vi "PH_Stepmotor_BaseClass.ProcCases.vi"(0 "i ref in":refnum<vi>, 1 "selector":string, 2 "Data":T1, 3 "call cluster":T2={"Object"="", "Selector"="", "CallType"=enum."synchronous", "Async Object"="", "Async Selector"="", "Data Descriptor"="", "Data"=[], "Error #"=0, "Expire"=0}, 5 "error in":errorcluster) -> (14 "i ref out":refnum<vi>, 17 "answer cluster":T2={"Object"="", "Selector"="", "CallType"=enum."synchronous", "Async Object"="", "Async Selector"="", "Data Descriptor"="", "Data"=[], "Error #"=0, "Expire"=0}, 19 "error out":errorcluster)   [LabVIEW 2014, in "PH_Stepmotor_BaseClass.lvlib"]
doc: "This method is called by a process from within the default case in the event loop. The methods of a class that are linked to events will be called from THIS method. Add your code here."
uses:
  PH_Stepmotor_BaseClass.lvlib
  CSCore/CSSystem/CoreDefs/CoreDefs.call_type.ctl
  CSCore/BaseProcess/BaseProcess.descriptor string definition.ctl
  CSCore/CSSystem/CoreDefs/CoreDefs.rawDataType.ctl
  PH_PSDBWriter/PH_PSDBWriter.Thread Commands.ctl
  PH_Stepmotor_BaseClass.Axis Settings.ctl
  PH_Stepmotor_BaseClass.Motor Type.ctl
  PH_Stepmotor_BaseClass.Axis Direction.ctl
  CSCore/CSSystem/CoreLib/CoreLib.string 2 byte array.vi
  CSCore/CSSystem/CoreLib/CoreLib.byte array 2 short.vi
  CSCore/CSSystem/CoreLib/CoreLib.byte array 2 int.vi
  CSCore/CSSystem/CoreLib/CoreLib.byte array 2 double.vi
  CSCore/CSSystem/CoreLib/CoreLib.byte array 2 string.vi
  CSCore/CSSystem/CoreLib/CoreLib.lvlib
  CSCore/BaseProcess/BaseProcess.lvlib
  PH_PSDBWriter/PH_PSDBWriter.lvlib
  CSCore/CAEObj/CAEObj.lvlib
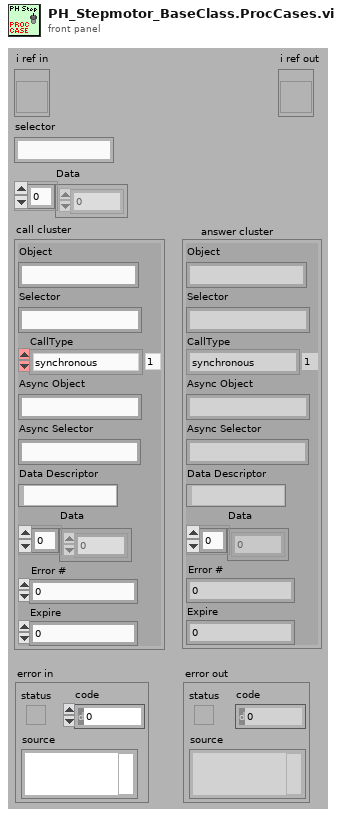
[diagram p1: front panel]
types:
  T1 = typedef "CoreDefs.rawDataType.ctl" = i8[]
  T2 = typedef "CoreDefs.call_type.ctl" = cluster{"Object":string, "Selector":string, "CallType":enum16{"simple", "synchronous", "asynchronous"}, "Async Object":string, "Async Selector":string, "Data Descriptor":T3, "Data":T1, "Error #":i32, "Expire":u32}
  T3 = typedef "BaseProcess.lvlib/BaseProcess.descriptor string definition.ctl" = string
  T4 = typedef "PH_Stepmotor_BaseClass.lvlib/PH_Stepmotor_BaseClass.Axis Settings.ctl" = cluster{"Sign change":bool, "Width":dbl, "Calibration":dbl, "Unit":string, "Motor Type":T5, "Unit Width":string, "Unit CF":string}
  T5 = typedef "PH_Stepmotor_BaseClass.lvlib/PH_Stepmotor_BaseClass.Motor Type.ctl" = enum16{"Unspecific", "OWIS 49.120.2633", "OWIS 49.060.1033", "OWIS 43.040.2558", "Diamond Motion 2200 series", "OWIS 49.120.266B.MV6", "Calorimeter", "Linear Stage 1", "MICOS VT-80", "MICOS VT-80 S", "Standa Rotstage nt0.95A", "PUF RA 320.200", "PUF RA 800.200", "PUF RA 800.400", "PUF RA 400.50", "1324.nn.800.50", "1324.n9c.800.50", "1324.nn.320.200", "1324.nn.400.200", "1324.nn.800.200", "1324.nn.400.50", "1324.8c9c.800.50", "1324.8c9c.400.200"}
  T6 = typedef "PH_Stepmotor_BaseClass.lvlib/PH_Stepmotor_BaseClass.Axis Direction.ctl" = enum16{"forward", "backward"}
  T7 = typedef "PH_PSDBWriter.lvlib/PH_PSDBWriter.PHELIX-Subsystems.ctl" = i32
  T8 = typedef "PH_PSDBWriter.lvlib/PH_PSDBWriter.Thread Commands.ctl" = u16
  T9 = typedef "PH_Stepmotor_BaseClass.lvlib/PH_Stepmotor_BaseClass.i attribute.ctl" = cluster{"Device Error":errorcluster, "Axes PSDB Thread":cluster{"Ref":refnum<vi>, "Q-Ref":refnum<queue>, "Data Status":T10}, "Axes":T11[], "Axes PSDB Infos":cluster{"GUI Name":string, "PSDB Instance ID":i32, "PSDB Status Service ID":i32, "Axis":i32, "Class":string}[], "GUI Refs":T14}
  T10 = typedef "PH_PSDBWriter.lvlib/PH_PSDBWriter.Data Status.ctl" = i16
  T11 = typedef "PH_Stepmotor_BaseClass.lvlib/PH_Stepmotor_BaseClass.Axis Attributes.ctl" = cluster{"Settings":T4, "Endswitch?":bool, "DIM Service IDs":T12, "Activity":T13, "Configured?":bool, "Position":cluster{"Current":i32, "Target":i32}, "Position to set":cluster{"New?":bool, "Wanted":i32}, "Stop?":bool, "Reset?":bool, "Move?":bool, "Nothing connected?":bool}
  T12 = typedef "PH_Stepmotor_BaseClass.lvlib/PH_Stepmotor_BaseClass.Axis DIM Service IDs.ctl" = cluster{"Settings":i32, "Information":i32}
  T13 = typedef "PH_Stepmotor_BaseClass.lvlib/PH_Stepmotor_BaseClass.Axis Activity.ctl" = enum16{"No Information", "stopped", "running", "Failure", "Alarm", "stopped at backward ES", "stopped at foreward ES"}
  T14 = typedef "PH_Stepmotor_BaseClass.lvlib/PH_Stepmotor_BaseClass.GUI Refs.ctl" = cluster{"Axes Configuration":refnum<vi>, "Device Error":refnum<vi>, "Axes PSDB Infos":refnum<vi>}
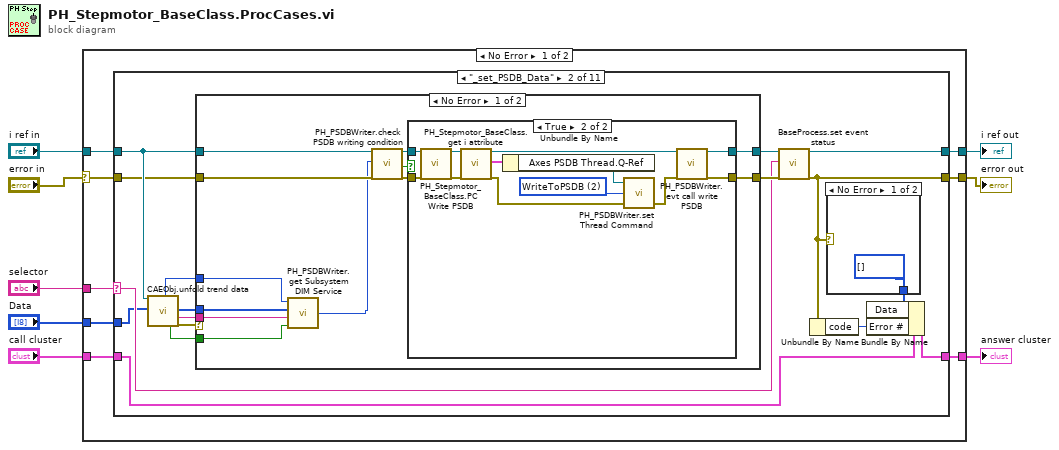
[diagram p0: block diagram]
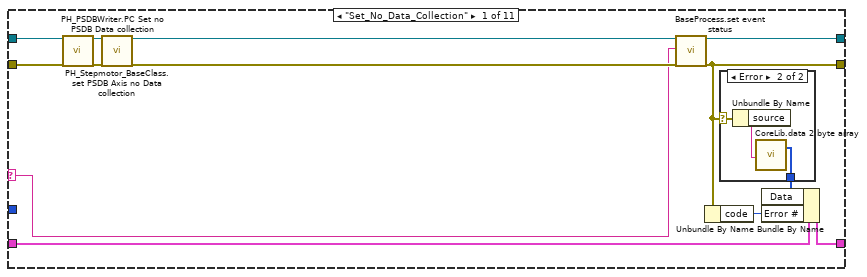
[diagram p2: hidden frame]
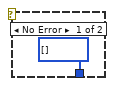
[diagram p3: hidden frame]
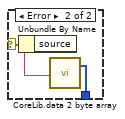
[diagram p6: hidden frame]
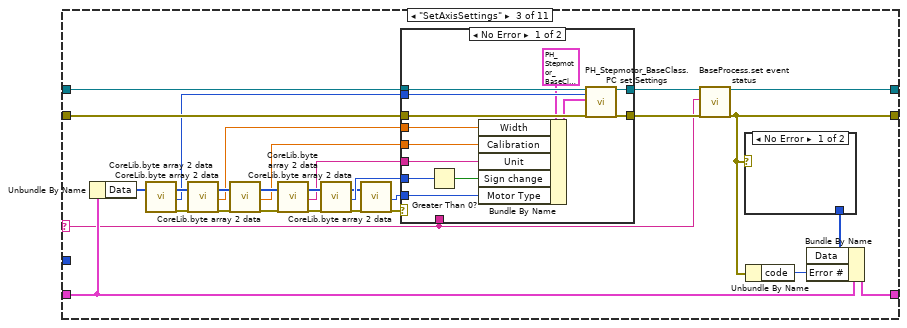
[diagram p7: hidden frame]
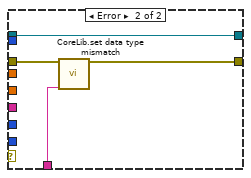
[diagram p8: hidden frame]
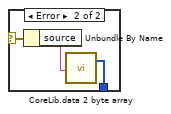
[diagram p9: hidden frame]
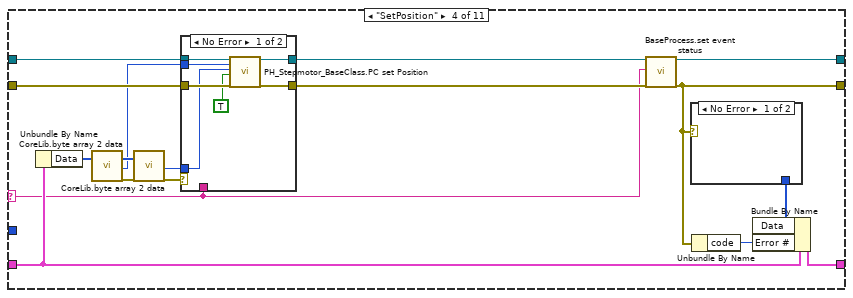
[diagram p10: hidden frame]
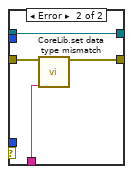
[diagram p11: hidden frame]
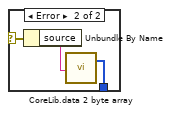
[diagram p12: hidden frame]
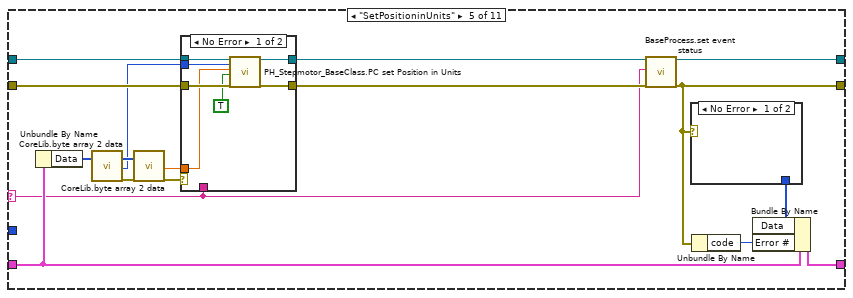
[diagram p13: hidden frame]
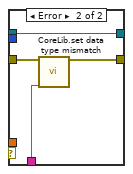
[diagram p14: hidden frame]
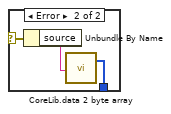
[diagram p15: hidden frame]
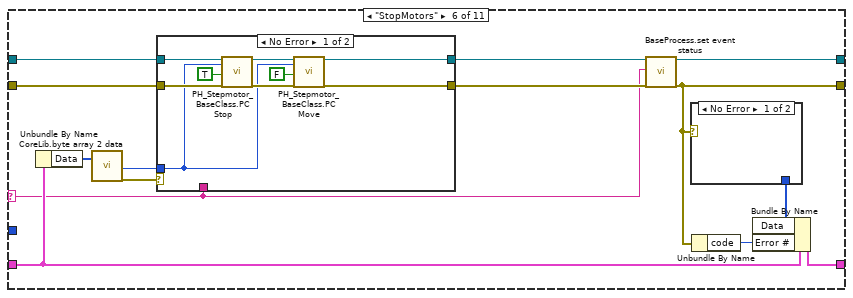
[diagram p16: hidden frame]
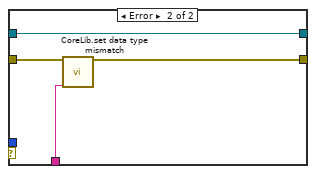
[diagram p17: hidden frame]
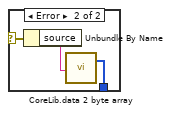
[diagram p18: hidden frame]
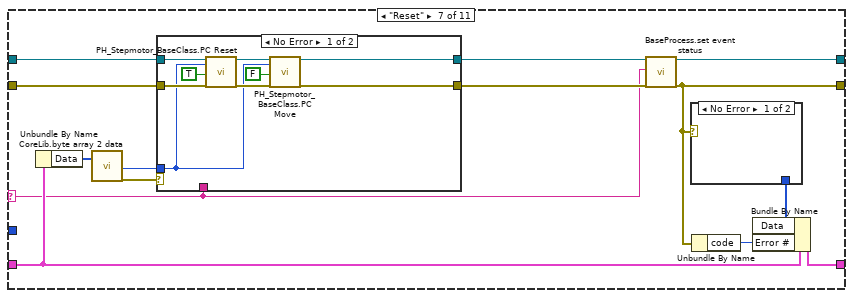
[diagram p19: hidden frame]
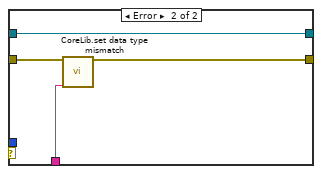
[diagram p20: hidden frame]
diagram:
  n1 = case shown="No Error" "error in" {
    selector: "error in" -> [w11 w342]
    tunnel: [w16 w341] -> w8
    tunnel: [w10 w342] -> w7
    tunnel: "call cluster" -> [w15 w341]
    tunnel: "selector" -> [w14 _]
    tunnel: [w9 w343] -> w4
    tunnel: "i ref in" -> [w13 w343]
    tunnel: "Data" -> [w12 _]
    frame No Error {
      n2 = case shown="\"_set_PSDB_Data\"" w14 {
        selector: w14 -> [w17 w35 w92 w135 w166 w196 w226 w259 w289 w319 w335]
        tunnel: [w26 w48 w109 w146 w177 w205 w235 w268 w298 w327 w337] -> w9
        tunnel: w15 -> [w29 w36 w93 w136 w167 w197 w227 w260 w290 w320 w333]
        tunnel: [w28 w50 w111 w148 w179 w207 w237 w270 w300 w329 w338] -> w16
        tunnel: w11 -> [w23 w39 w94 w137 w168 w198 w228 w261 w291 w321 w340]
        tunnel: [w25 w47 w108 w145 w176 w204 w234 w267 w297 w326 w339] -> w10
        tunnel: w13 -> [w22 w40 w106 w143 w174 w202 w232 w265 w295 w324 w336]
        tunnel: w12 -> [_ w34 _ _ _ _ _ _ _ _ w334]
        frame "Set_No_Data_Collection" {
          n3 = call "PH_PSDBWriter.PC Set no PSDB Data collection.vi"("i ref in"=w22, "error IO"=w23) -> ("i ref out"=w19:refnum<vi>, "error out"=w21:errorcluster)  [unwired: 16 in]
          n4 = call "PH_Stepmotor_BaseClass.set PSDB Axis no Data collection.vi"("i ref in"=w19, "error in"=w21) -> ("i ref out"=w18:refnum<vi>, "error out"=w20:errorcluster)  [unwired: 16 in]
          n5 = call "BaseProcess.set event status.vi"("i ref in"=w18, "EventStatus"=w17, "error in (no error)"=w20) -> ("i ref out"=w26:refnum<vi>, "error out"=w25:errorcluster)  [unwired: 14 in, 1 out]
          n6 = Unbundle By Name(w25) -> ("code"=w27:i32)
          n7 = case shown="Error" w25 {
            selector: w25 -> [_ w33]
            tunnel: [T1 [] ("byteArray out") w31] -> w24
            frame No Error {
            }
            frame Error {
              n8 = Unbundle By Name(w33) -> ("source"=w32:string)
              n9 = call-poly "CoreLib.data 2 byte array.vi"("string"=w32) -> ("byteArray out"=w31:T1)  [unwired: 18 in]
            }
          }
          n10 = Bundle By Name(cluster=w29, "Data"=w24, "Error #"=w27) -> (w28:T2)
        }
        frame "_set_PSDB_Data" {
          n11 = call "CAEObj.unfold trend data.vi"("i ref in"=w40, "raw trend data"=w34) -> ("quality"=w41:i32, "no link"=w44:bool, "data"=w42:i8[], "typeDescriptor"=w43:string, "error out"=w45:errorcluster)  [unwired: 9 in, 4 out]
          n12 = case shown="No Error" w45 {
            tunnel: w39 -> [w62 w78]
            tunnel: [w61 w77] -> w38
            tunnel: [w60 w78] -> w37
            tunnel: w40 -> [w58 w77]
            tunnel: w44 -> [w52 _]
            tunnel: w43 -> [w54 _]
            tunnel: w42 -> [w55 _]
            tunnel: w41 -> [w53 _]
            frame No Error {
              n13 = call "PH_PSDBWriter.get Subsystem DIM Service.vi"("no link"=w52, "typeDescriptor"=w54, "data"=w55, "quality"=w53) -> ("PHELIX Subsystems"=w51:T7)
              n14 = call "PH_PSDBWriter.check PSDB writing condition.vi"("i ref in"=w58, "wanted Subsystem"=w51, "error IO"=w62) -> ("i ref out"=w57:refnum<vi>, "write PSDB?"=w56:bool, "error out"=w59:errorcluster)  [unwired: 14 in]
              n15 = case shown="True" w56 {
                tunnel: w59 -> [w63 w76]
                tunnel: [w64 w67] -> w61
                tunnel: [w63 w65] -> w60
                tunnel: w57 -> [w64 w75]
                frame False {
                }
                frame True {
                  w71 = T8 2 items=["None", "GetInstanceID", "WriteToPSDB"] ("PSDB Thread Command")
                  n16 = call "PH_Stepmotor_BaseClass.PC Write PSDB.vi"("i ref in"=w75, "error IO"=w76) -> ("i ref out"=w69:refnum<vi>, "error out"=w70:errorcluster)  [unwired: 16 in]
                  n17 = call "PH_Stepmotor_BaseClass.get i attribute.vi"("i ref in"=w69, "error in (no error)"=w70) -> ("i ref out"=w68:refnum<vi>, "i attribute"=w73:T9, "error out"=w74:errorcluster)  [unwired: 15 in]
                  n18 = Unbundle By Name(w73) -> ("Axes PSDB Thread.Q-Ref"=w72:refnum<queue>)
                  n19 = call "PH_PSDBWriter.set Thread Command.vi"("error in (no error)"=w74, "PSDB Thread Command"=w71, "Queue in"=w72) -> ("error out"=w66:errorcluster)  [unwired: 2 in]
                  n20 = call "PH_PSDBWriter.evt call write PSDB.vi"("i ref in"=w68, "error in (no error)"=w66) -> ("i ref out"=w67:refnum<vi>, "error out"=w65:errorcluster)  [unwired: 16 in]
                }
              }
            }
            frame Error {
            }
          }
          n21 = call "BaseProcess.set event status.vi"("i ref in"=w38, "EventStatus"=w35, "error in (no error)"=w37) -> ("i ref out"=w48:refnum<vi>, "error out"=w47:errorcluster)  [unwired: 14 in, 1 out]
          n22 = Unbundle By Name(w47) -> ("code"=w49:i32)
          n23 = case shown="No Error" w47 {
            selector: w47 -> [_ w82]
            tunnel: [T1 [] ("byteArray out") w80] -> w46
            frame No Error {
            }
            frame Error {
              n24 = Unbundle By Name(w82) -> ("source"=w81:string)
              n25 = call-poly "CoreLib.data 2 byte array.vi"("string"=w81) -> ("byteArray out"=w80:T1)  [unwired: 18 in]
            }
          }
          n26 = Bundle By Name(cluster=w36, "Data"=w46, "Error #"=w49) -> (w50:T2)
        }
        frame "SetAxisSettings" {
          n27 = Unbundle By Name(w93) -> ("Data"=w99:T1)
          n28 = call-poly "CoreLib.byte array 2 data.vi"("byteArray"=w99) -> ("byteArray out"=w103:T1, "i32"=w91:i32, "error out"=w102:errorcluster)  [unwired: 16 in]
          n29 = call-poly "CoreLib.byte array 2 data.vi"("byteArray"=w103, "error in (no error)"=w102) -> ("byteArray out"=w101:T1, "d64"=w87:dbl, "error out"=w100:errorcluster)  [unwired: 15 in]
          n30 = call-poly "CoreLib.byte array 2 data.vi"("byteArray"=w101, "error in (no error)"=w100) -> ("byteArray out"=w97:T1, "d64"=w88:dbl, "error out"=w96:errorcluster)  [unwired: 15 in]
          n31 = call-poly "CoreLib.byte array 2 data.vi"("byteArray"=w97, "error in (no error)"=w96) -> ("byteArray out"=w98:T1, "string"=w89:string, "error out"=w95:errorcluster)  [unwired: 15 in]
          n32 = call-poly "CoreLib.byte array 2 data.vi"("byteArray"=w98, "error in (no error)"=w95) -> ("byteArray out"=w86:T1, "i16"=w90:i16, "error out"=w85:errorcluster)  [unwired: 15 in]
          n33 = call-poly "CoreLib.byte array 2 data.vi"("byteArray"=w86, "error in (no error)"=w85) -> ("i16"=w83:i16, "error out"=w84:errorcluster)  [unwired: 15 in, 1 out]
          n34 = case shown="No Error" w84 {
            tunnel: w106 -> [w124 w125]
            tunnel: [w123 w125] -> w105
            tunnel: [w122 w127] -> w104
            tunnel: w94 -> [w121 w128]
            tunnel: w92 -> [_ w126]
            tunnel: w91 -> [w120 _]
            tunnel: w90 -> [w116 _]
            tunnel: w89 -> [w114 _]
            tunnel: w88 -> [w113 _]
            tunnel: w87 -> [w112 _]
            tunnel: w83 -> [w117 _]
            frame No Error {
              n35 = Greater Than 0?(x=w116) -> (x > 0?=w115:bool)
              n36 = Bundle By Name(cluster=T4 {"Sign change"=FALSE, "Width"=0.0, "Calibration"=0.0, "Unit"="Steps", "Motor Type"=enum."Unspecific", "Unit Width"="", "Unit CF"=""} ("Settings to set"), "Width"=w112, "Calibration"=w113, "Unit"=w114, "Sign change"=w115, "Motor Type"=w117) -> (w118:T4)
              n37 = call "PH_Stepmotor_BaseClass.PC set Settings.vi"("i ref in"=w124, "axis"=w120, "Settings to set"=w118, "error in (no error)"=w121) -> ("i ref out"=w123:refnum<vi>, "error out"=w122:errorcluster)  [unwired: 14 in]
            }
            frame Error {
              n38 = call "CoreLib.set data type mismatch.vi"("error in (no error)"=w128, "error source"=w126) -> ("error out"=w127:errorcluster)  [unwired: 17 in]
            }
          }
          n39 = call "BaseProcess.set event status.vi"("i ref in"=w105, "EventStatus"=w92, "error in (no error)"=w104) -> ("i ref out"=w109:refnum<vi>, "error out"=w108:errorcluster)  [unwired: 14 in, 1 out]
          n40 = case shown="No Error" w108 {
            selector: w108 -> [_ w131]
            tunnel: [_ w130] -> w107
            frame No Error {
            }
            frame Error {
              n41 = Unbundle By Name(w131) -> ("source"=w129:string)
              n42 = call-poly "CoreLib.data 2 byte array.vi"("string"=w129) -> ("byteArray out"=w130:T1)  [unwired: 18 in]
            }
          }
          n43 = Unbundle By Name(w108) -> ("code"=w110:i32)
          n44 = Bundle By Name(cluster=w93, "Data"=w107, "Error #"=w110) -> (w111:T2)
        }
        frame "SetPosition" {
          n45 = Unbundle By Name(w136) -> ("Data"=w138:T1)
          n46 = call-poly "CoreLib.byte array 2 data.vi"("byteArray"=w138) -> ("byteArray out"=w140:T1, "i32"=w134:i32, "error out"=w139:errorcluster)  [unwired: 16 in]
          n47 = call-poly "CoreLib.byte array 2 data.vi"("byteArray"=w140, "error in (no error)"=w139) -> ("i32"=w133:i32, "error out"=w132:errorcluster)  [unwired: 15 in, 1 out]
          n48 = case shown="No Error" w132 {
            tunnel: w143 -> [w155 w156]
            tunnel: [w154 w156] -> w142
            tunnel: [w153 w158] -> w141
            tunnel: w137 -> [w152 w159]
            tunnel: w135 -> [_ w157]
            tunnel: w134 -> [w151 _]
            tunnel: w133 -> [w150 _]
            frame No Error {
              n49 = call "PH_Stepmotor_BaseClass.PC set Position.vi"("i ref in"=w155, "axis"=w151, "Position to set"=w150, "Set?"=TRUE, "error in (no error)"=w152) -> ("i ref out"=w154:refnum<vi>, "error out"=w153:errorcluster)  [unwired: 12 in, 1 out]
            }
            frame Error {
              n50 = call "CoreLib.set data type mismatch.vi"("error in (no error)"=w159, "error source"=w157) -> ("error out"=w158:errorcluster)  [unwired: 17 in]
            }
          }
          n51 = call "BaseProcess.set event status.vi"("i ref in"=w142, "EventStatus"=w135, "error in (no error)"=w141) -> ("i ref out"=w146:refnum<vi>, "error out"=w145:errorcluster)  [unwired: 14 in, 1 out]
          n52 = case shown="No Error" w145 {
            selector: w145 -> [_ w162]
            tunnel: [_ w161] -> w144
            frame No Error {
            }
            frame Error {
              n53 = Unbundle By Name(w162) -> ("source"=w160:string)
              n54 = call-poly "CoreLib.data 2 byte array.vi"("string"=w160) -> ("byteArray out"=w161:T1)  [unwired: 18 in]
            }
          }
          n55 = Unbundle By Name(w145) -> ("code"=w147:i32)
          n56 = Bundle By Name(cluster=w136, "Data"=w144, "Error #"=w147) -> (w148:T2)
        }
        frame "SetPositioninUnits" {
          n57 = Unbundle By Name(w167) -> ("Data"=w169:T1)
          n58 = call-poly "CoreLib.byte array 2 data.vi"("byteArray"=w169) -> ("byteArray out"=w171:T1, "i32"=w165:i32, "error out"=w170:errorcluster)  [unwired: 16 in]
          n59 = call-poly "CoreLib.byte array 2 data.vi"("byteArray"=w171, "error in (no error)"=w170) -> ("d64"=w164:dbl, "error out"=w163:errorcluster)  [unwired: 15 in, 1 out]
          n60 = case shown="No Error" w163 {
            tunnel: w174 -> [w186 w187]
            tunnel: [w185 w187] -> w173
            tunnel: [w184 w189] -> w172
            tunnel: w168 -> [w183 w190]
            tunnel: w166 -> [_ w188]
            tunnel: w165 -> [w182 _]
            tunnel: w164 -> [w181 _]
            frame No Error {
              n61 = call "PH_Stepmotor_BaseClass.PC set Position in Units.vi"("i ref in"=w186, "axis"=w182, "Position to set [Units]"=w181, "Set?"=TRUE, "error in (no error)"=w183) -> ("i ref out"=w185:refnum<vi>, "error out"=w184:errorcluster)  [unwired: 12 in, 1 out]
            }
            frame Error {
              n62 = call "CoreLib.set data type mismatch.vi"("error in (no error)"=w190, "error source"=w188) -> ("error out"=w189:errorcluster)  [unwired: 17 in]
            }
          }
          n63 = call "BaseProcess.set event status.vi"("i ref in"=w173, "EventStatus"=w166, "error in (no error)"=w172) -> ("i ref out"=w177:refnum<vi>, "error out"=w176:errorcluster)  [unwired: 14 in, 1 out]
          n64 = case shown="No Error" w176 {
            selector: w176 -> [_ w193]
            tunnel: [_ w192] -> w175
            frame No Error {
            }
            frame Error {
              n65 = Unbundle By Name(w193) -> ("source"=w191:string)
              n66 = call-poly "CoreLib.data 2 byte array.vi"("string"=w191) -> ("byteArray out"=w192:T1)  [unwired: 18 in]
            }
          }
          n67 = Unbundle By Name(w176) -> ("code"=w178:i32)
          n68 = Bundle By Name(cluster=w167, "Data"=w175, "Error #"=w178) -> (w179:T2)
        }
        frame "StopMotors" {
          n69 = Unbundle By Name(w197) -> ("Data"=w199:T1)
          n70 = call-poly "CoreLib.byte array 2 data.vi"("byteArray"=w199) -> ("i32"=w195:i32, "error out"=w194:errorcluster)  [unwired: 16 in, 1 out]
          n71 = case shown="No Error" w194 {
            tunnel: w202 -> [w216 w217]
            tunnel: [w210 w217] -> w201
            tunnel: [w212 w219] -> w200
            tunnel: w198 -> [w214 w220]
            tunnel: w196 -> [_ w218]
            tunnel: w195 -> [w209 _]
            frame No Error {
              n72 = call "PH_Stepmotor_BaseClass.PC Stop.vi"("i ref in"=w216, "axis"=w209, "Stop"=TRUE, "error in (no error)"=w214) -> ("i ref out"=w211:refnum<vi>, "error out"=w215:errorcluster)  [unwired: 14 in]
              n73 = call "PH_Stepmotor_BaseClass.PC Move.vi"("i ref in"=w211, "axis"=w209, "Move"=FALSE, "error in (no error)"=w215) -> ("i ref out"=w210:refnum<vi>, "error out"=w212:errorcluster)  [unwired: 14 in]
            }
            frame Error {
              n74 = call "CoreLib.set data type mismatch.vi"("error in (no error)"=w220, "error source"=w218) -> ("error out"=w219:errorcluster)  [unwired: 17 in]
            }
          }
          n75 = call "BaseProcess.set event status.vi"("i ref in"=w201, "EventStatus"=w196, "error in (no error)"=w200) -> ("i ref out"=w205:refnum<vi>, "error out"=w204:errorcluster)  [unwired: 14 in, 1 out]
          n76 = case shown="No Error" w204 {
            selector: w204 -> [_ w223]
            tunnel: [_ w222] -> w203
            frame No Error {
            }
            frame Error {
              n77 = Unbundle By Name(w223) -> ("source"=w221:string)
              n78 = call-poly "CoreLib.data 2 byte array.vi"("string"=w221) -> ("byteArray out"=w222:T1)  [unwired: 18 in]
            }
          }
          n79 = Unbundle By Name(w204) -> ("code"=w206:i32)
          n80 = Bundle By Name(cluster=w197, "Data"=w203, "Error #"=w206) -> (w207:T2)
        }
        frame "Reset" {
          n81 = Unbundle By Name(w227) -> ("Data"=w229:T1)
          n82 = call-poly "CoreLib.byte array 2 data.vi"("byteArray"=w229) -> ("i32"=w225:i32, "error out"=w224:errorcluster)  [unwired: 16 in, 1 out]
          n83 = case shown="No Error" w224 {
            tunnel: w232 -> [w246 w247]
            tunnel: [w240 w247] -> w231
            tunnel: [w242 w249] -> w230
            tunnel: w228 -> [w244 w250]
            tunnel: w226 -> [_ w248]
            tunnel: w225 -> [w239 _]
            frame No Error {
              n84 = call "PH_Stepmotor_BaseClass.PC Reset.vi"("i ref in"=w246, "axis"=w239, "Reset?"=TRUE ("Stop"), "error in (no error)"=w244) -> ("i ref out"=w241:refnum<vi>, "error out"=w245:errorcluster)  [unwired: 14 in]
              n85 = call "PH_Stepmotor_BaseClass.PC Move.vi"("i ref in"=w241, "axis"=w239, "Move"=FALSE, "error in (no error)"=w245) -> ("i ref out"=w240:refnum<vi>, "error out"=w242:errorcluster)  [unwired: 14 in]
            }
            frame Error {
              n86 = call "CoreLib.set data type mismatch.vi"("error in (no error)"=w250, "error source"=w248) -> ("error out"=w249:errorcluster)  [unwired: 17 in]
            }
          }
          n87 = call "BaseProcess.set event status.vi"("i ref in"=w231, "EventStatus"=w226, "error in (no error)"=w230) -> ("i ref out"=w235:refnum<vi>, "error out"=w234:errorcluster)  [unwired: 14 in, 1 out]
          n88 = case shown="No Error" w234 {
            selector: w234 -> [_ w253]
            tunnel: [_ w252] -> w233
            frame No Error {
            }
            frame Error {
              n89 = Unbundle By Name(w253) -> ("source"=w251:string)
              n90 = call-poly "CoreLib.data 2 byte array.vi"("string"=w251) -> ("byteArray out"=w252:T1)  [unwired: 18 in]
            }
          }
          n91 = Unbundle By Name(w234) -> ("code"=w236:i32)
          n92 = Bundle By Name(cluster=w227, "Data"=w233, "Error #"=w236) -> (w237:T2)
        }
        frame "AbsoluteMove" {
          n93 = Unbundle By Name(w260) -> ("Data"=w262:T1)
          n94 = call-poly "CoreLib.byte array 2 data.vi"("byteArray"=w262) -> ("byteArray out"=w255:T1, "i32"=w258:i32, "error out"=w257:errorcluster)  [unwired: 16 in]
          n95 = call-poly "CoreLib.byte array 2 data.vi"("byteArray"=w255, "error in (no error)"=w257) -> ("d64"=w254:dbl, "error out"=w256:errorcluster)  [unwired: 15 in, 1 out]
          n96 = case shown="No Error" w256 {
            tunnel: w265 -> [w276 w277]
            tunnel: [w275 w277] -> w264
            tunnel: [w274 w279] -> w263
            tunnel: w261 -> [w273 w280]
            tunnel: w259 -> [_ w278]
            tunnel: w258 -> [w272 _]
            tunnel: w254 -> [w271 _]
            frame No Error {
              n97 = call "PH_Stepmotor_BaseClass.PC Absolute Move.vi"("i ref in"=w276, "axis"=w272, "Target (Unit)"=w271, "error in (no error)"=w273) -> ("i ref out"=w275:refnum<vi>, "error out"=w274:errorcluster)  [unwired: 14 in]
            }
            frame Error {
              n98 = call "CoreLib.set data type mismatch.vi"("error in (no error)"=w280, "error source"=w278) -> ("error out"=w279:errorcluster)  [unwired: 17 in]
            }
          }
          n99 = call "BaseProcess.set event status.vi"("i ref in"=w264, "EventStatus"=w259, "error in (no error)"=w263) -> ("i ref out"=w268:refnum<vi>, "error out"=w267:errorcluster)  [unwired: 14 in, 1 out]
          n100 = case shown="No Error" w267 {
            selector: w267 -> [_ w283]
            tunnel: [_ w282] -> w266
            frame No Error {
            }
            frame Error {
              n101 = Unbundle By Name(w283) -> ("source"=w281:string)
              n102 = call-poly "CoreLib.data 2 byte array.vi"("string"=w281) -> ("byteArray out"=w282:T1)  [unwired: 18 in]
            }
          }
          n103 = Unbundle By Name(w267) -> ("code"=w269:i32)
          n104 = Bundle By Name(cluster=w260, "Data"=w266, "Error #"=w269) -> (w270:T2)
        }
        frame "RelativeMove" {
          n105 = Unbundle By Name(w290) -> ("Data"=w292:T1)
          n106 = call-poly "CoreLib.byte array 2 data.vi"("byteArray"=w292) -> ("byteArray out"=w285:T1, "i32"=w288:i32, "error out"=w287:errorcluster)  [unwired: 16 in]
          n107 = call-poly "CoreLib.byte array 2 data.vi"("byteArray"=w285, "error in (no error)"=w287) -> ("i16"=w284:i16, "error out"=w286:errorcluster)  [unwired: 15 in, 1 out]
          n108 = case shown="No Error" w286 {
            tunnel: w295 -> [w310 w311]
            tunnel: [w309 w311] -> w294
            tunnel: [w308 w313] -> w293
            tunnel: w291 -> [w307 w314]
            tunnel: w289 -> [_ w312]
            tunnel: w288 -> [w306 _]
            tunnel: w284 -> [w305 _]
            frame No Error {
              n109 = Equal To 0?(x=w305) -> (x = 0?=w304:bool)
              n110 = Select(t=PH_Stepmotor_BaseClass.Axis_Direction."forward", s=w304, f=PH_Stepmotor_BaseClass.Axis_Direction."backward" ("Direction")) -> (s? t:f=w302:T6)
              n111 = call "PH_Stepmotor_BaseClass.PC Relative Move.vi"("i ref in"=w310, "axis"=w306, "Direction"=w302, "error in (no error)"=w307) -> ("i ref out"=w309:refnum<vi>, "error out"=w308:errorcluster)  [unwired: 14 in]
            }
            frame Error {
              n112 = call "CoreLib.set data type mismatch.vi"("error in (no error)"=w314, "error source"=w312) -> ("error out"=w313:errorcluster)  [unwired: 17 in]
            }
          }
          n113 = call "BaseProcess.set event status.vi"("i ref in"=w294, "EventStatus"=w289, "error in (no error)"=w293) -> ("i ref out"=w298:refnum<vi>, "error out"=w297:errorcluster)  [unwired: 14 in, 1 out]
          n114 = case shown="No Error" w297 {
            selector: w297 -> [_ w317]
            tunnel: [_ w316] -> w296
            frame No Error {
            }
            frame Error {
              n115 = Unbundle By Name(w317) -> ("source"=w315:string)
              n116 = call-poly "CoreLib.data 2 byte array.vi"("string"=w315) -> ("byteArray out"=w316:T1)  [unwired: 18 in]
            }
          }
          n117 = Unbundle By Name(w297) -> ("code"=w299:i32)
          n118 = Bundle By Name(cluster=w290, "Data"=w296, "Error #"=w299) -> (w300:T2)
        }
        frame "ClearError" {
          n119 = call "PH_Stepmotor_BaseClass.set Device Error.vi"("i ref in"=w324, "Device Error"=errorcluster {"status"=FALSE, "code"=0, "source"=""}, "error in"=w321) -> ("i ref out"=w323:refnum<vi>, "error out"=w322:errorcluster)  [unwired: 15 in]
          n120 = call "BaseProcess.set event status.vi"("i ref in"=w323, "EventStatus"=w319, "error in (no error)"=w322) -> ("i ref out"=w327:refnum<vi>, "error out"=w326:errorcluster)  [unwired: 14 in, 1 out]
          n121 = case shown="No Error" w326 {
            selector: w326 -> [_ w332]
            tunnel: [_ w331] -> w325
            frame No Error {
            }
            frame Error {
              n122 = Unbundle By Name(w332) -> ("source"=w330:string)
              n123 = call-poly "CoreLib.data 2 byte array.vi"("string"=w330) -> ("byteArray out"=w331:T1)  [unwired: 18 in]
            }
          }
          n124 = Unbundle By Name(w326) -> ("code"=w328:i32)
          n125 = Bundle By Name(cluster=w320, "Data"=w325, "Error #"=w328) -> (w329:T2)
        }
        frame Default {
          n126 = call "PH_PSDBWriter.ProcCases.vi"("i ref in"=w336, "selector"=w335, "Data"=w334, "call cluster"=w333, "error in"=w340) -> ("i ref out"=w337:refnum<vi>, "answer cluster"=w338:T2, "error out"=w339:errorcluster)  [unwired: 12 in]
        }
      }
    }
    frame Error {
    }
  }
  "answer cluster" <- w8
  "i ref out" <- w4
  "error out" <- w7
